vi "Shot Overlay 3 (SubVI).vi"(6 "Image Out":T1, 7 "Particle Measurements (Pixels) (Particle Analysis 1)":dbl[][](array[numeric]), 8 "Particle Measurements (Real-World) (Particle Analysis 1)":dbl[][](array[numeric]), 9 "Nb Circles (Circle Detection 1)":i32) -> (1 "Player area overlay":T1, 2 "Player Position Pixels":dbl[][](array[numeric]), 3 "Puck position pixels":dbl[][](array[numeric]))   [LabVIEW 2013]
uses:
  <vilib>/vision/Image Controls.llb/IMAQ Image.ctl
panel:
  out "Particle Measurements (Real-World) (Particle Analysis 1) 2":dbl[][](array[numeric])
  out "output cluster":cluster{i32, i32, i32, i32}
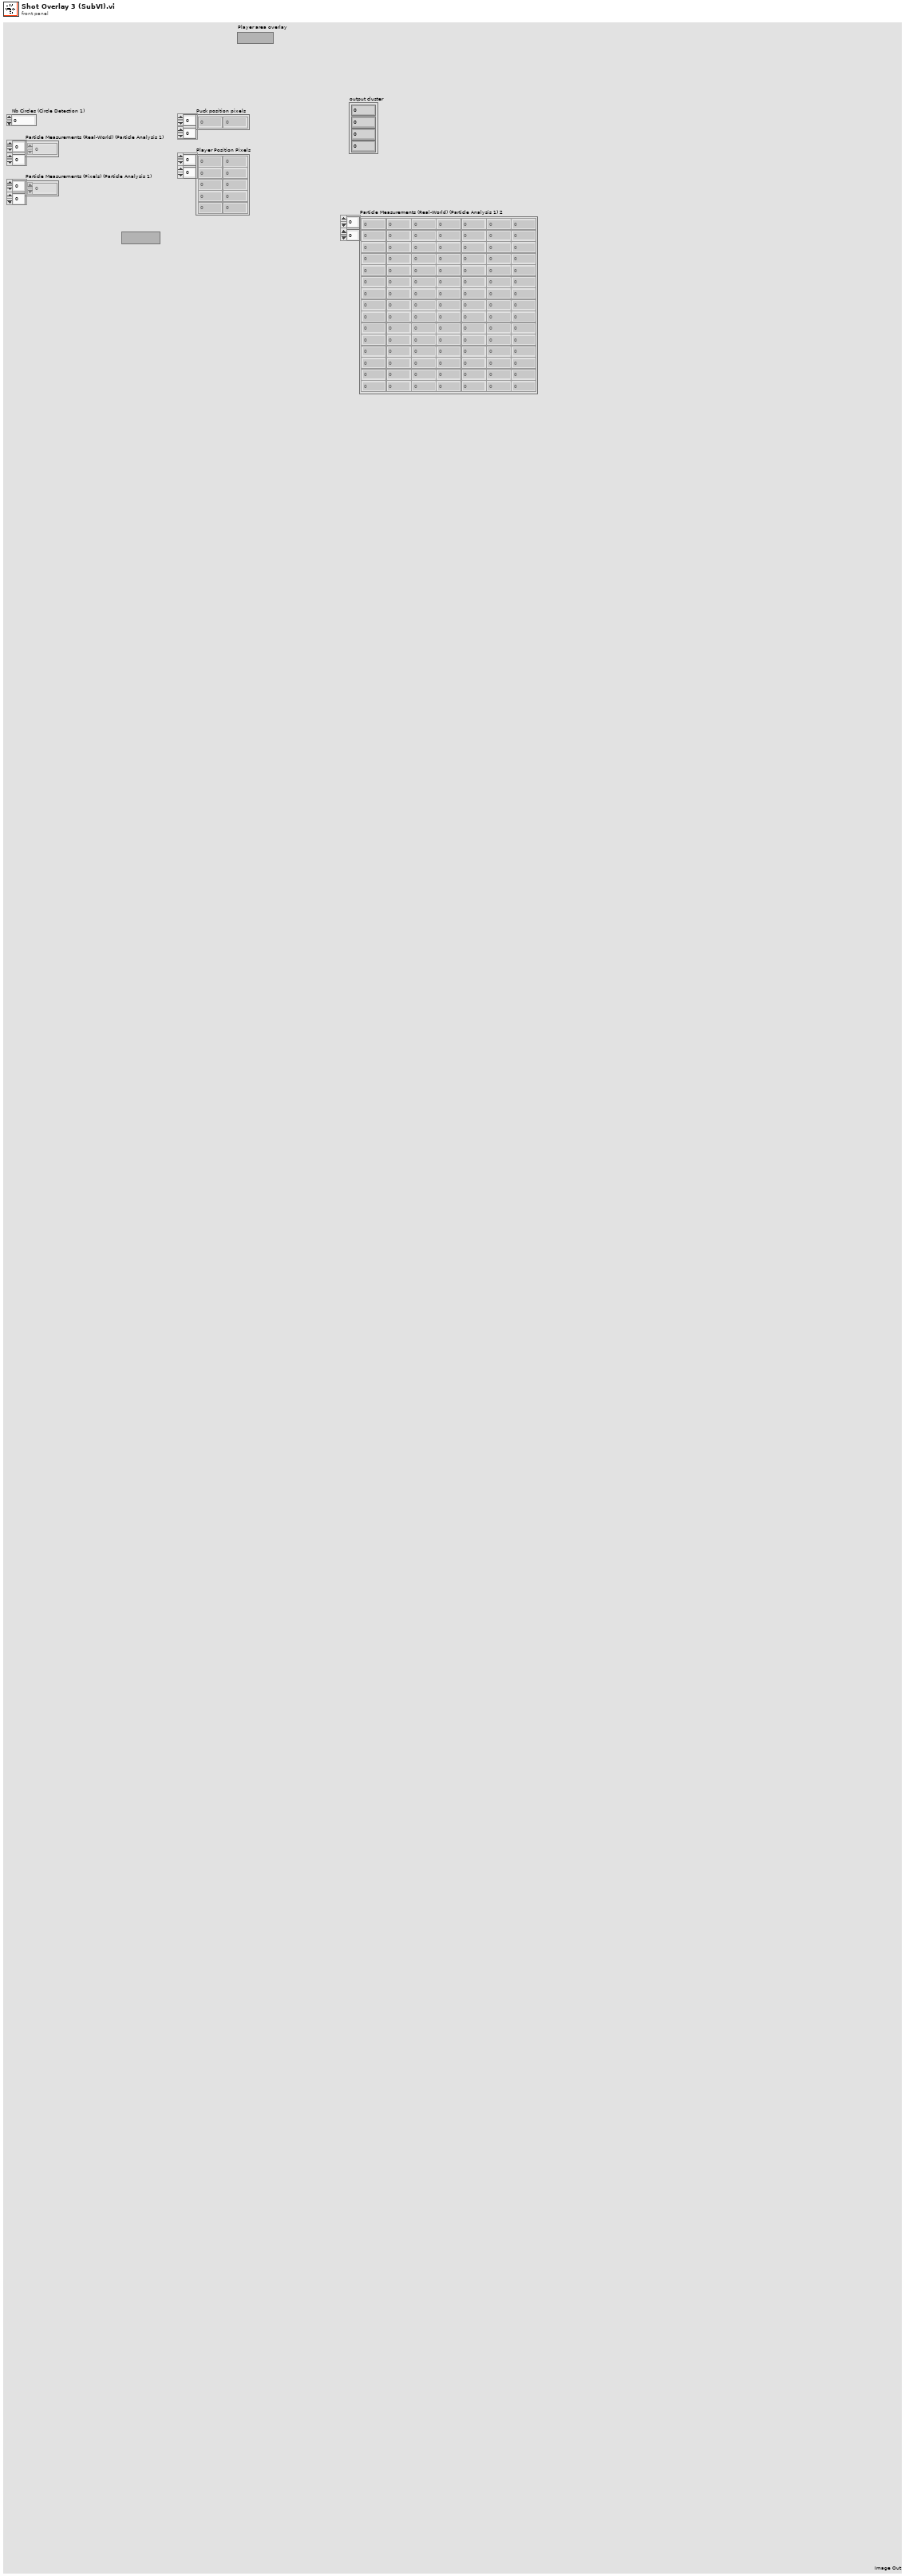
[diagram p1: front panel]
types:
  T1 = typedef "IMAQ Image.ctl" = refnum<image>
  T2 = cluster{"Desired Font (Application)":enum16{"User-specified Font", "Application Font", "System Font", "Dialog Font"}, "[User-specified Font]":cluster{"Font Name":string, "Size":i16, "Strikeout?":bool, "Italic?":bool, "Underline?":bool, "Outline?":bool, "Shadow?":bool, "Bold?":bool, "Rotation Angle":dbl}, "Horizontal Alignment":i16, "Vertical Alignment":i16}
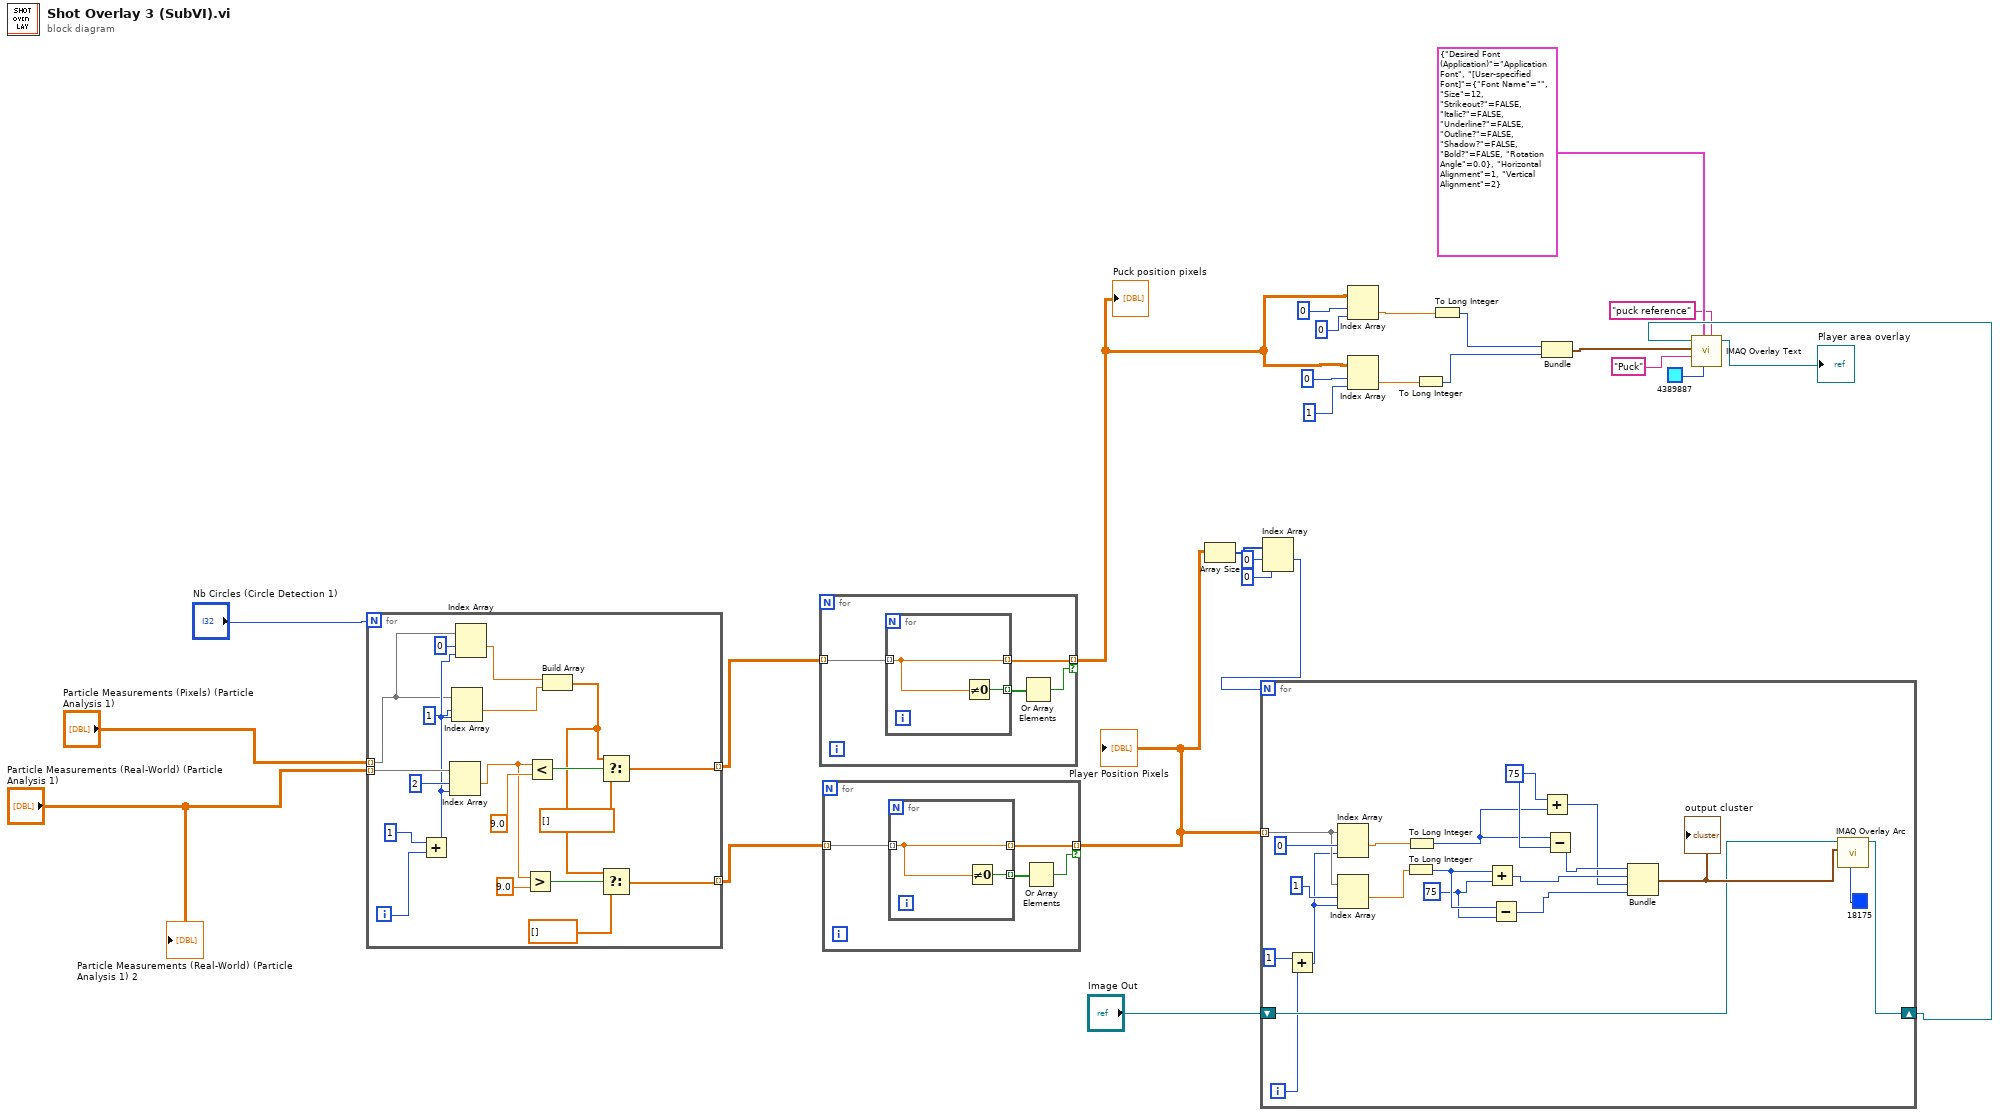
[diagram p0: block diagram]
diagram:
  n1 = for {
    N: "Nb Circles (Circle Detection 1)" -> [_]
    tunnel: "Particle Measurements (Real-World) (Particle Analysis 1)" -> [w40] mode=indexing
    tunnel: [w42] -> w24 mode=indexing
    tunnel: [w29] -> w25 mode=indexing
    tunnel: "Particle Measurements (Pixels) (Particle Analysis 1)" -> [w28] mode=indexing
    i -> [w46]
    n2 = Add(x=1, y=w46) -> (x+y=w38:i32)
    n3 = Index Array(array=w40, index #1=2 ("index"), index #2=w38) -> (element #1=w33:dbl)  [unwired: 1 out]
    n4 = Index Array(array=w28, index #1=1 ("index"), index #2=w38) -> (element #1=w36:dbl)  [unwired: 1 out]
    n5 = Index Array(array=w28, index #1=0 ("index"), index #2=w38) -> (element #1=w37:dbl)  [unwired: 1 out]
    n6 = Greater?(x=w33, y=9.0) -> (0:w32:bool)
    n7 = Less?(x=w33, y=9.0) -> (x < y?=w43:bool)
    n8 = Build Array(w37, w36) -> (w31:dbl[])
    n9 = Select(t=w31, s=w43, f=dbl[] []) -> (s? t:f=w42:dbl[])
    n10 = Select(t=w31, s=w32, f=dbl[] []) -> (s? t:f=w29:dbl[])
  }
  n11 = for {
    tunnel: w24 -> [w51] mode=indexing
    tunnel: [w49] -> w12 mode=indexing if=w48
    n12 = for {
      tunnel: w51 -> [w52] mode=indexing
      tunnel: [w53] -> w50 mode=indexing
      tunnel: [w52] -> w49 mode=indexing
      n13 = Not Equal To 0?(x=w52) -> (x != 0?=w53:bool)
    }
    n14 = Or Array Elements(Boolean array=w50) -> (logical OR=w48:bool)
  }
  "Puck position pixels" <- w12
  n15 = for {
    tunnel: w25 -> [w57] mode=indexing
    tunnel: [w55] -> w18 mode=indexing if=w54
    n16 = for {
      tunnel: w57 -> [w58] mode=indexing
      tunnel: [w59] -> w56 mode=indexing
      tunnel: [w58] -> w55 mode=indexing
      n17 = Not Equal To 0?(x=w58) -> (x != 0?=w59:bool)
    }
    n18 = Or Array Elements(Boolean array=w56) -> (logical OR=w54:bool)
  }
  "Player Position Pixels" <- w18
  n19 = Array Size(array=w18) -> (size(s)=w21:i32[])
  n20 = Index Array(array=w21, index #1=0 ("index"), index #2=0 ("index")) -> (element #1=w17:i32)  [unwired: 1 out]
  n21 = for {
    N: w17 -> [_]
    tunnel: w18 -> [w63] mode=indexing
    shift-right: [w67] -> w6
    shift-left: "Image Out" -> [w68]
    i -> [w65]
    w75 = 75 ("y")
    w79 = 75 ("x")
    n22 = Add(x=1, y=w65) -> (x+y=w61:i32)
    n23 = Index Array(array=w63, index #1=0 ("index"), index #2=w61) -> (element #1=w78:dbl)  [unwired: 1 out]
    n24 = Index Array(array=w63, index #1=1 ("index"), index #2=w61) -> (element #1=w60:dbl)  [unwired: 1 out]
    n25 = To Long Integer(number=w60) -> (32bit integer=w76:i32)
    n26 = To Long Integer(number=w78) -> (32bit integer=w77:i32)
    n27 = Add(x=w76, y=w75) -> (x+y=w73:i32)
    n28 = Subtract(x=w76, y=w75) -> (x-y=w71:i32)
    n29 = Add(x=w79, y=w77) -> (x+y=w72:i32)
    n30 = Subtract(x=w77, y=w79) -> (x-y=w74:i32)
    n31 = Bundle(w74, w73, w72, w71) -> (w69:cluster{i32, i32, i32, i32})  [unwired: 1 in]
    "output cluster" <- w69
    n32 = call "IMAQ Overlay Arc"("Color"=u32 18175, "Bounding Rectangle"=w69, "Image"=w68) -> ("Image Out"=w67:T1)  [unwired: 7 in, 1 out]
  }
  n33 = Index Array(array=w12, index (row)=0, index (col)=0 ("disabled index (col)")) -> (element=w11:dbl)
  n34 = Index Array(array=w12, index (row)=0 ("index"), index (col)=1 ("disabled index (col)")) -> (element=w10:dbl)
  n35 = To Long Integer(number=w10) -> (32bit integer=w8:i32)
  n36 = To Long Integer(number=w11) -> (32bit integer=w9:i32)
  n37 = Bundle(w9, w8) -> (w7:cluster{i32, i32})  [unwired: 1 in]
  n38 = call "IMAQ Overlay Text"("Group"="puck reference", "Text Color (black)"=u32 4389887, "Font, Size & Style"=T2 {"Desired Font (Application)"=enum."Application Font", "[User-specified Font]"={"Font Name"="", "Size"=12, "Strikeout?"=FALSE, "Italic?"=FALSE, "Underline?"=FALSE, "Outline?"=FALSE, "Shadow?"=FALSE, "Bold?"=FALSE, "Rotation Angle"=0.0}, "Horizontal Alignment"=1, "Vertical Alignment"=2}, "String"="Puck", "Origin"=w7, "Image"=w6) -> ("Image Out"=→"Player area overlay":T1)  [unwired: 4 in, 1 out]
  "Particle Measurements (Real-World) (Particle Analysis 1) 2" <- "Particle Measurements (Real-World) (Particle Analysis 1)"
